vi "odometry test.vi"() -> ()   [LabVIEW 2017]
panel:
  out "XY Graph":cluster{"X":dbl, "Y":dbl}[](graph)
  in  "stop":bool
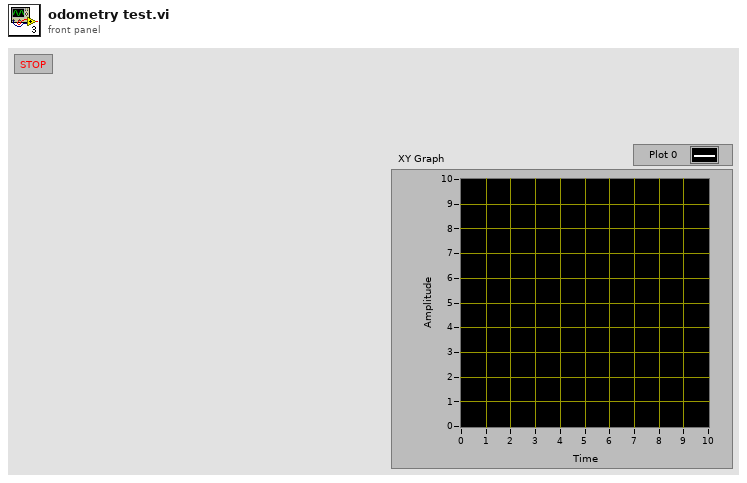
[diagram p1: front panel]
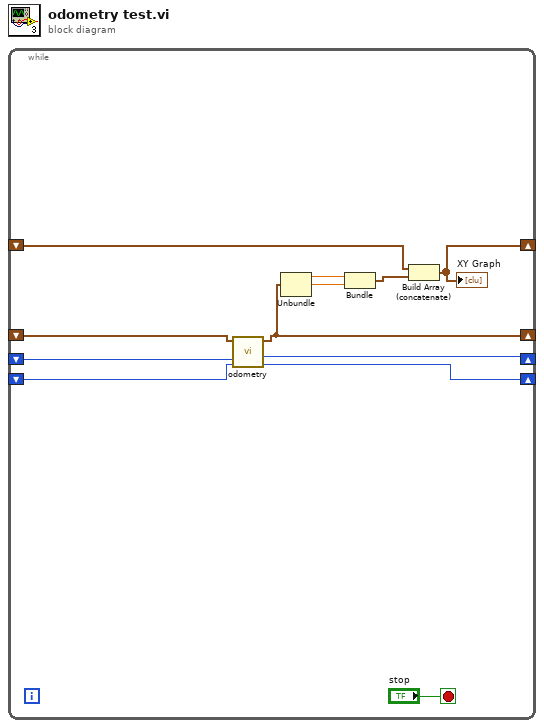
[diagram p0: block diagram]
diagram:
  n1 = while {
    shift-right: [w6] -> _
    shift-left: _ -> [w11]
    shift-right: [w9] -> _
    shift-left: _ -> [w10]
    shift-right: [w8] -> _
    shift-left: _ -> [w7]
    shift-right: [w1] -> _
    shift-left: _ -> [w2]
    stop <- "stop" stop-if-true
    n2 = call "odometry.vi"("ENCB in"=w7, "ENCA in"=w10, "Position"=w11) -> ("ENCB OUT"=w8:i32, "ENCA OUT"=w9:i32, "X, Y, BEARING"=w6:cluster{dbl, dbl, dbl})  [unwired: 5 in]
    n3 = Unbundle(w6) -> (w5:dbl, w4:dbl)  [unwired: 1 out]
    n4 = Bundle(w5, w4) -> (w3:cluster{dbl, dbl})  [unwired: 1 in]
    n5 = Build Array (concatenate)(w2, w3) -> (w1:cluster{dbl, dbl}[])
    "XY Graph" <- w1
  }
